vi "Meas Config Panel - Sample Rate Selectors Update.vi"(8 "error in (no error)":errorcluster, 11 "tab control ref":refnum<vi>) -> (0 "error out":errorcluster, 3 "sampling rate":T1)   [LabVIEW 2020]
doc: "Updates sample rate selectors, return calculated sampling rate for selected page (mode)."
uses:
  Meas Sampling Rate Mode.ctl
  drivers/DMM/3458A Sampling Rate.ctl
  drivers/AWG/AWG Clock Setup Mode.ctl
  drivers/AWG/AWG.lvlib
  drivers/DMM/3458A Virtual Digitizer.lvlib
panel:
  in  "fs mode":T3 caption="Sampling rate mode"
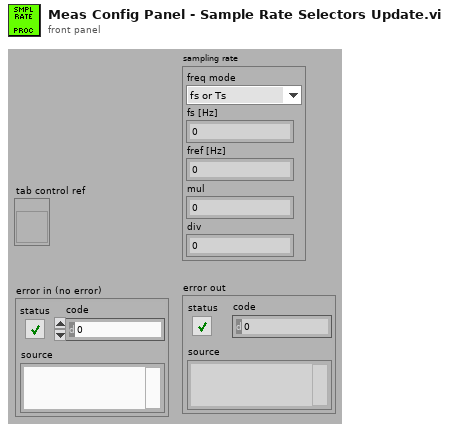
[diagram p1: front panel]
types:
  T1 = typedef "3458A Virtual Digitizer.lvlib/3458A Sampling Rate.ctl" = cluster{"freq mode":T2, "fs [Hz]":dbl, "fref [Hz]":dbl, "mul":dbl, "div":dbl}
  T2 = typedef "AWG.lvlib/AWG Clock Setup Mode.ctl" = enum16{"fs or Ts", "fs or Ts with fref", "fref/N", "fref*M/N", "fref*Ratio"}
  T3 = typedef "Meas Sampling Rate Mode.ctl" = enum16{"Frequency", "Period"}
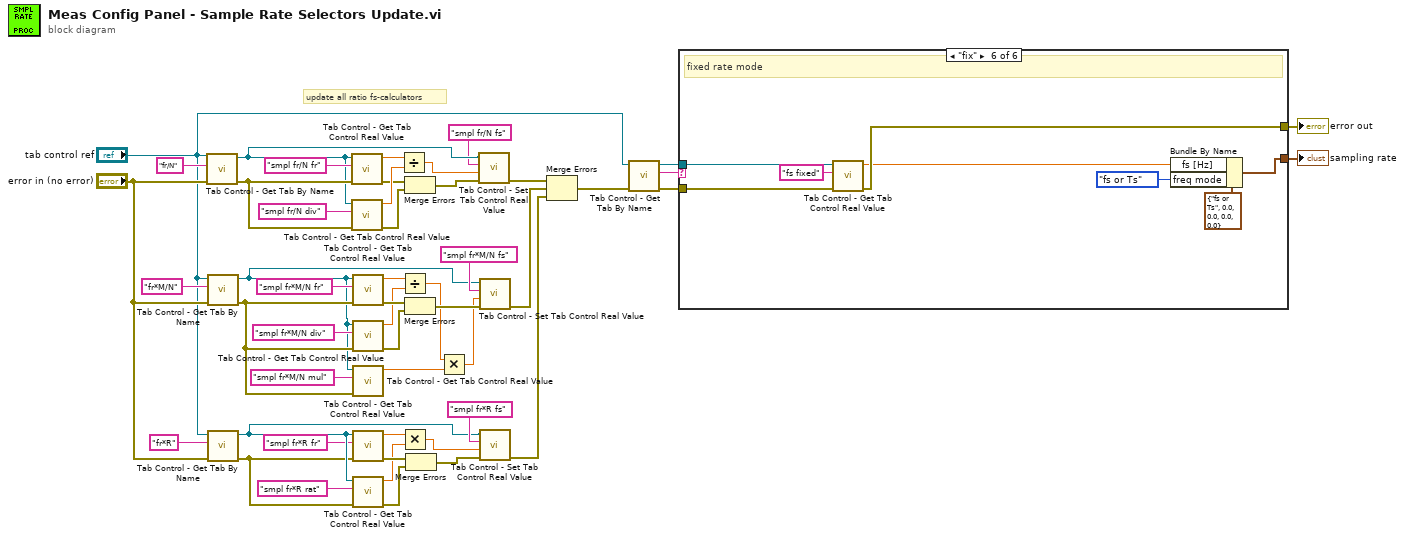
[diagram p0: block diagram]
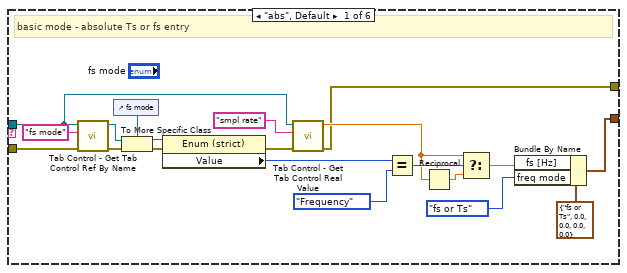
[diagram p2: hidden frame]
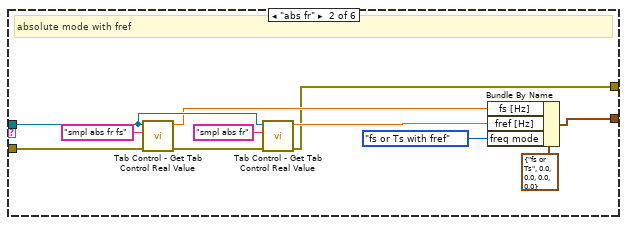
[diagram p3: hidden frame]
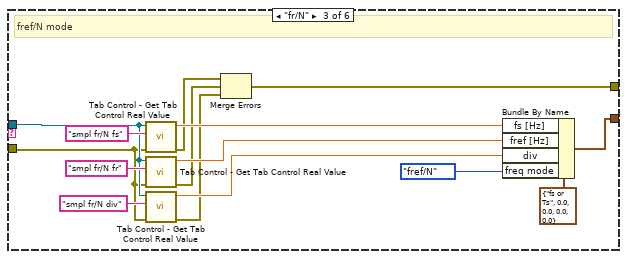
[diagram p4: hidden frame]
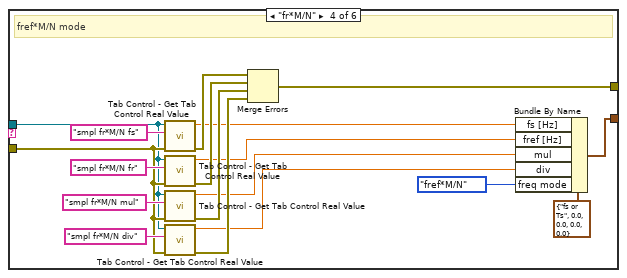
[diagram p5: hidden frame]
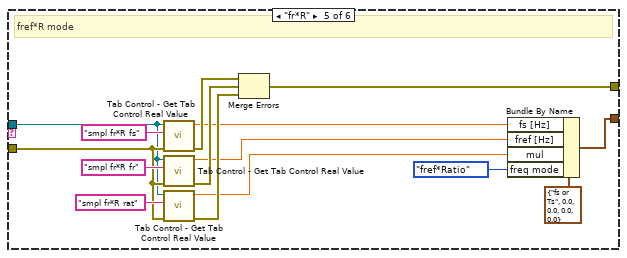
[diagram p6: hidden frame]
diagram:
  # "update all ratio fs-calculators"
  n1 = call "Tab Control - Get Tab By Name.vi"("error in (no error)"="error in (no error)", "page caption (empty)"="fr/N", "page control ref"="tab control ref") -> ("error out"=w47:errorcluster, "page ref out"=w40:refnum<vi>)  [unwired: 6 in, 1 out]
  n2 = call "Tab Control - Get Tab By Name.vi"("error in (no error)"="error in (no error)", "page caption (empty)"="fr*M/N", "page control ref"="tab control ref") -> ("error out"=w28:errorcluster, "page ref out"=w27:refnum<vi>)  [unwired: 6 in, 1 out]
  n3 = call "Tab Control - Get Tab By Name.vi"("error in (no error)"="error in (no error)", "page caption (empty)"="fr*R", "page control ref"="tab control ref") -> ("error out"=w15:errorcluster, "page ref out"=w22:refnum<vi>)  [unwired: 6 in, 1 out]
  n4 = call "Tab Control - Get Tab Control Real Value.vi"("error in (no error)"=w47, "control label"="smpl fr/N fr", "page ref"=w40) -> ("error out"=w43:errorcluster, "value"=w46:dbl)  [unwired: 7 in]
  n5 = call "Tab Control - Get Tab Control Real Value.vi"("error in (no error)"=w47, "control label"="smpl fr/N div", "page ref"=w40) -> ("error out"=w44:errorcluster, "value"=w45:dbl)  [unwired: 7 in]
  n6 = call "Tab Control - Get Tab Control Real Value.vi"("error in (no error)"=w28, "control label"="smpl fr*M/N fr", "page ref"=w27) -> ("error out"=w36:errorcluster, "value"=w33:dbl)  [unwired: 7 in]
  n7 = call "Tab Control - Get Tab Control Real Value.vi"("error in (no error)"=w28, "control label"="smpl fr*M/N div", "page ref"=w27) -> ("error out"=w35:errorcluster, "value"=w34:dbl)  [unwired: 7 in]
  n8 = call "Tab Control - Get Tab Control Real Value.vi"("error in (no error)"=w28, "control label"="smpl fr*M/N mul", "page ref"=w27) -> ("value"=w26:dbl)  [unwired: 7 in, 1 out]
  n9 = call "Tab Control - Get Tab Control Real Value.vi"("error in (no error)"=w15, "control label"="smpl fr*R fr", "page ref"=w22) -> ("error out"=w19:errorcluster, "value"=w16:dbl)  [unwired: 7 in]
  n10 = call "Tab Control - Get Tab Control Real Value.vi"("error in (no error)"=w15, "control label"="smpl fr*R rat", "page ref"=w22) -> ("error out"=w18:errorcluster, "value"=w17:dbl)  [unwired: 7 in]
  n11 = Divide(x=w46, y=w45) -> (x/y=w41:dbl)
  n12 = Divide(x=w33, y=w34) -> (x/y=w25:dbl)
  n13 = Multiply(x=w16, y=w17) -> (x*y=w21:dbl)
  n14 = Merge Errors(w43, w44) -> (w42:errorcluster)
  n15 = Merge Errors(w36, w35) -> (w37:errorcluster)
  n16 = Merge Errors(w19, w18) -> (w20:errorcluster)
  n17 = Multiply(x=w25, y=w26) -> (x*y=w24:dbl)
  n18 = call "Tab Control - Set Tab Control Real Value.vi"("error in (no error)"=w42, "value"=w41, "control label"="smpl fr/N fs", "page ref"=w40) -> ("error out"=w10:errorcluster)  [unwired: 7 in]
  n19 = call "Tab Control - Set Tab Control Real Value.vi"("error in (no error)"=w37, "value"=w24, "control label"="smpl fr*M/N fs", "page ref"=w27) -> ("error out"=w9:errorcluster)  [unwired: 7 in]
  n20 = call "Tab Control - Set Tab Control Real Value.vi"("error in (no error)"=w20, "value"=w21, "control label"="smpl fr*R fs", "page ref"=w22) -> ("error out"=w8:errorcluster)  [unwired: 7 in]
  n21 = Merge Errors(w10, w9, w8) -> (w7:errorcluster)
  n22 = call "Tab Control - Get Tab By Name.vi"("error in (no error)"=w7, "page control ref"="tab control ref") -> ("error out"=w5:errorcluster, "page caption out"=w6:string, "page ref out"=w4:refnum<vi>)  [unwired: 7 in]
  n23 = case shown="\"fix\"" w6 {
    tunnel: [w66 w80 w95 w113 w127 w136] -> w1
    tunnel: w5 -> [w64 w78 w89 w104 w120 w134]
    tunnel: w4 -> [w55 w74 w90 w103 w119 w133]
    tunnel: [w52 w71 w82 w97 w115 w131] -> w2
    frame "abs", Default {
      # "basic mode - absolute Ts or fs entry"
      n24 = call "Tab Control - Get Tab Control Ref By Name.vi"("error in (no error)"=w64, "control label"="fs mode", "page ref"=w55) -> ("error out"=w63:errorcluster, "control ref out"=w62:refnum<vi>)  [unwired: 7 in]
      n25 = control-ref of="fs mode"() -> (w61:refnum<vi>)
      n26 = To More Specific Class(target class=w61, reference=w62, error in=w63) -> (specific class reference=w58:refnum<vi>, error out=w59:errorcluster)
      n27 = property class="Enum (strict)"(reference=w58, error in=w59) -> (error out=w56:errorcluster, "Value"=w57:T3)  [unwired: 1 out]
      n28 = call "Tab Control - Get Tab Control Real Value.vi"("error in (no error)"=w56, "control label"="smpl rate", "page ref"=w55) -> ("error out"=w52:errorcluster, "value"=w53:dbl)  [unwired: 7 in]
      n29 = Equal?(x=w57, y=Meas_Sampling_Rate_Mode."Frequency") -> (x = y?=w69:bool)
      n30 = Reciprocal(x=w53) -> (1/x=w70:dbl)
      n31 = Select(t=w53, s=w69, f=w70) -> (s? t:f=w67:dbl)
      n32 = Bundle By Name(cluster=T1 {"freq mode"=enum."fs or Ts", "fs [Hz]"=0.0, "fref [Hz]"=0.0, "mul"=0.0, "div"=0.0} ("sampling rate"), "fs [Hz]"=w67, "freq mode"=AWG_Clock_Setup_Mode."fs or Ts") -> (w66:T1)
    }
    frame "abs fr" {
      # "absolute mode with fref"
      n33 = call "Tab Control - Get Tab Control Real Value.vi"("error in (no error)"=w78, "control label"="smpl abs fr fs", "page ref"=w74) -> ("error out"=w75:errorcluster, "value"=w73:dbl)  [unwired: 7 in]
      n34 = call "Tab Control - Get Tab Control Real Value.vi"("error in (no error)"=w75, "control label"="smpl abs fr", "page ref"=w74) -> ("error out"=w71:errorcluster, "value"=w72:dbl)  [unwired: 7 in]
      n35 = Bundle By Name(cluster=T1 {"freq mode"=enum."fs or Ts", "fs [Hz]"=0.0, "fref [Hz]"=0.0, "mul"=0.0, "div"=0.0} ("sampling rate"), "fs [Hz]"=w73, "fref [Hz]"=w72, "freq mode"=AWG_Clock_Setup_Mode."fs or Ts with fref") -> (w80:T1)
    }
    frame "fr/N" {
      # "fref/N mode"
      n36 = call "Tab Control - Get Tab Control Real Value.vi"("error in (no error)"=w89, "control label"="smpl fr/N fs", "page ref"=w90) -> ("error out"=w85:errorcluster, "value"=w88:dbl)  [unwired: 7 in]
      n37 = call "Tab Control - Get Tab Control Real Value.vi"("error in (no error)"=w89, "control label"="smpl fr/N fr", "page ref"=w90) -> ("error out"=w84:errorcluster, "value"=w87:dbl)  [unwired: 7 in]
      n38 = call "Tab Control - Get Tab Control Real Value.vi"("error in (no error)"=w89, "control label"="smpl fr/N div", "page ref"=w90) -> ("error out"=w83:errorcluster, "value"=w86:dbl)  [unwired: 7 in]
      n39 = Merge Errors(w85, w84, w83) -> (w82:errorcluster)
      n40 = Bundle By Name(cluster=T1 {"freq mode"=enum."fs or Ts", "fs [Hz]"=0.0, "fref [Hz]"=0.0, "mul"=0.0, "div"=0.0} ("sampling rate"), "fs [Hz]"=w88, "fref [Hz]"=w87, "div"=w86, "freq mode"=AWG_Clock_Setup_Mode."fref/N") -> (w95:T1)
    }
    frame "fr*M/N" {
      # "fref*M/N mode"
      n41 = call "Tab Control - Get Tab Control Real Value.vi"("error in (no error)"=w104, "control label"="smpl fr*M/N fs", "page ref"=w103) -> ("error out"=w111:errorcluster, "value"=w101:dbl)  [unwired: 7 in]
      n42 = call "Tab Control - Get Tab Control Real Value.vi"("error in (no error)"=w104, "control label"="smpl fr*M/N fr", "page ref"=w103) -> ("error out"=w110:errorcluster, "value"=w100:dbl)  [unwired: 7 in]
      n43 = call "Tab Control - Get Tab Control Real Value.vi"("error in (no error)"=w104, "control label"="smpl fr*M/N mul", "page ref"=w103) -> ("error out"=w109:errorcluster, "value"=w99:dbl)  [unwired: 7 in]
      n44 = call "Tab Control - Get Tab Control Real Value.vi"("error in (no error)"=w104, "control label"="smpl fr*M/N div", "page ref"=w103) -> ("error out"=w102:errorcluster, "value"=w98:dbl)  [unwired: 7 in]
      n45 = Merge Errors(w111, w110, w109, w102) -> (w97:errorcluster)
      n46 = Bundle By Name(cluster=T1 {"freq mode"=enum."fs or Ts", "fs [Hz]"=0.0, "fref [Hz]"=0.0, "mul"=0.0, "div"=0.0} ("sampling rate"), "fs [Hz]"=w101, "fref [Hz]"=w100, "mul"=w99, "div"=w98, "freq mode"=AWG_Clock_Setup_Mode."fref*M/N") -> (w113:T1)
    }
    frame "fr*R" {
      # "fref*R mode"
      n47 = call "Tab Control - Get Tab Control Real Value.vi"("error in (no error)"=w120, "control label"="smpl fr*R fs", "page ref"=w119) -> ("error out"=w123:errorcluster, "value"=w118:dbl)  [unwired: 7 in]
      n48 = call "Tab Control - Get Tab Control Real Value.vi"("error in (no error)"=w120, "control label"="smpl fr*R fr", "page ref"=w119) -> ("error out"=w122:errorcluster, "value"=w117:dbl)  [unwired: 7 in]
      n49 = call "Tab Control - Get Tab Control Real Value.vi"("error in (no error)"=w120, "control label"="smpl fr*R rat", "page ref"=w119) -> ("error out"=w121:errorcluster, "value"=w116:dbl)  [unwired: 7 in]
      n50 = Merge Errors(w123, w122, w121) -> (w115:errorcluster)
      n51 = Bundle By Name(cluster=T1 {"freq mode"=enum."fs or Ts", "fs [Hz]"=0.0, "fref [Hz]"=0.0, "mul"=0.0, "div"=0.0} ("sampling rate"), "fs [Hz]"=w118, "fref [Hz]"=w117, "mul"=w116, "freq mode"=AWG_Clock_Setup_Mode."fref*Ratio") -> (w127:T1)
    }
    frame "fix" {
      # "fixed rate mode"
      n52 = call "Tab Control - Get Tab Control Real Value.vi"("error in (no error)"=w134, "control label"="fs fixed", "page ref"=w133) -> ("error out"=w131:errorcluster, "value"=w130:dbl)  [unwired: 7 in]
      n53 = Bundle By Name(cluster=T1 {"freq mode"=enum."fs or Ts", "fs [Hz]"=0.0, "fref [Hz]"=0.0, "mul"=0.0, "div"=0.0} ("sampling rate"), "fs [Hz]"=w130, "freq mode"=AWG_Clock_Setup_Mode."fs or Ts") -> (w136:T1)
    }
  }
  "error out" <- w2
  "sampling rate" <- w1
